vi "volumeStartInfo.vi"(6 "scan min":T3, 7 "scan max":T3, 8 "scan specification":T4={"x amplitude"=1000, "x resolution (pixels)"=28, "x offset fly-forward (iterations)"=50, "x offset fly-back (iterations)"=100, "y resolution (nr. of lines)"=80, "y step size"=30, "iterations per pixel"=5, "number of frames"=-1, "y offset (pixels)"=0, "number of y-brake lines  (before y-fly-back)"=0, "number y-brake lines (after y-fly-back)"=40, "number of y-fly-back steps"=0, "lines per z step"=1, "number of z/intensity tuples"=228, "number of repetitions (volumes or planes)"=-1, "z step size derived"=32, "choose the beginning of z scan"=FALSE, "number of frames (settings)"=80, "FPGA trajectory?"=TRUE, "Pockels cell voltage (bits)"=0, "Vy min(bits)"=0, "Vz min(bits)"=0}, 11 "derived values":T2) -> (3 "volume info":T1)   [LabVIEW 2010]
uses:
  scan_specification_cluster.ctl
  derived_values_cluster.ctl
panel:
  in  "set vol from scan settings":bool
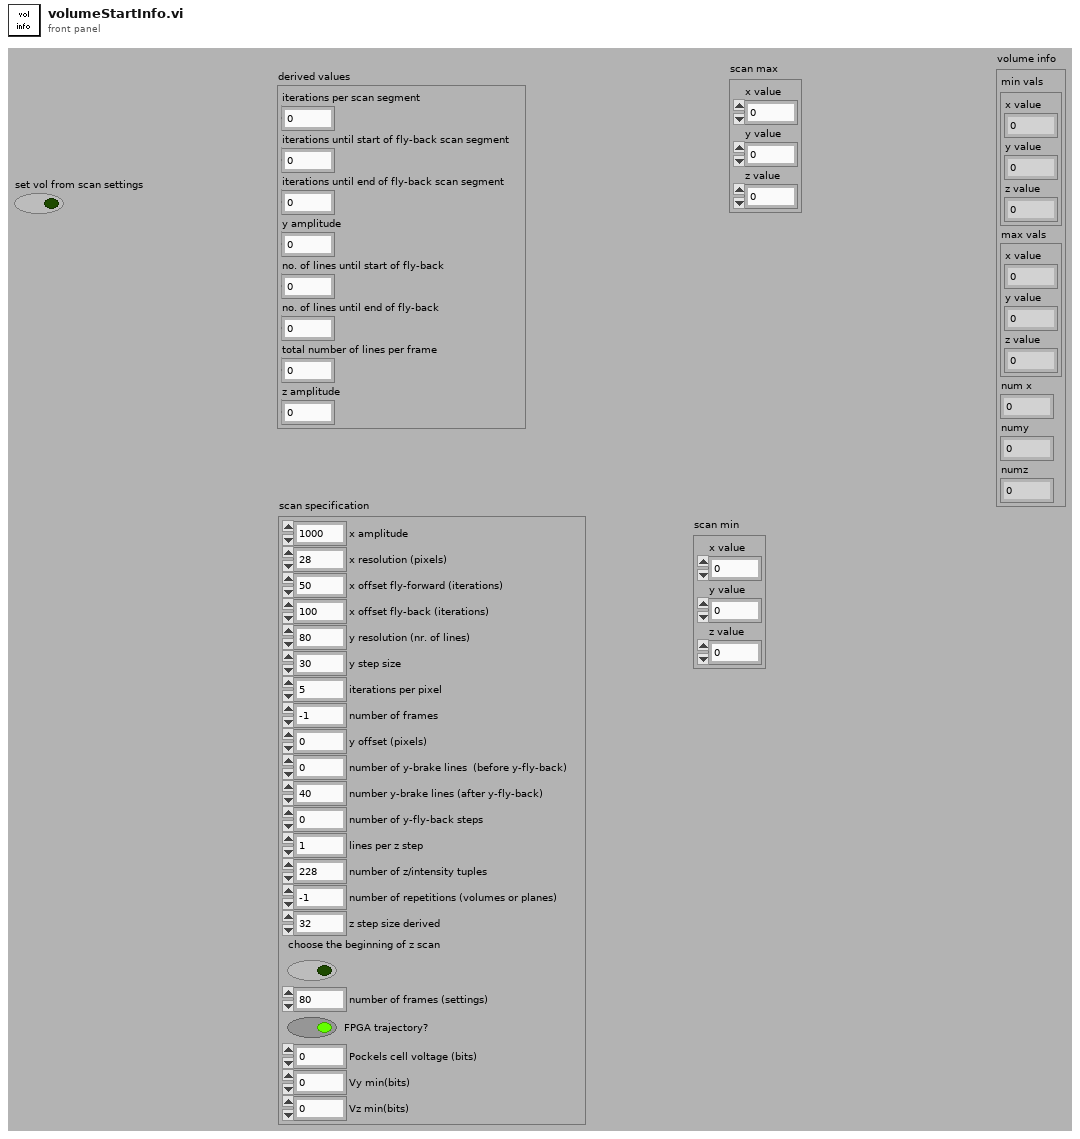
[diagram p1: front panel]
types:
  T1 = cluster{"min vals":cluster{"x value":i16, "y value":i16, "z value":i16}, "max vals":cluster{"x value":i16, "y value":i16, "z value":i16}, "num x":u32, "numy":u32, "numz":u32}
  T2 = typedef "derived_values_cluster.ctl" = cluster{"iterations per scan segment":u16, "iterations until start of fly-back scan segment":u16, "iterations until end of fly-back scan segment":u16, "y amplitude":u16, "no. of lines until start of fly-back":u16, "no. of lines until end of fly-back":u16, "total number of lines per frame ":u16, "z amplitude":u16}
  T3 = cluster{"x value":i16, "y value":i16, "z value":i16}
  T4 = typedef "scan_specification_cluster.ctl" = cluster{"x amplitude":u16, "x resolution (pixels)":u16, "x offset fly-forward (iterations)":u16, "x offset fly-back (iterations)":u16, "y resolution (nr. of lines)":u16, "y step size":u16, "iterations per pixel":u16, "number of frames":i32, "y offset (pixels)":u16, "number of y-brake lines  (before y-fly-back)":u16, "number y-brake lines (after y-fly-back)":u16, "number of y-fly-back steps":u16, "lines per z step":u16, "number of z/intensity tuples":u16, "number of repetitions (volumes or planes)":i32, "z step size derived":u16, "choose the beginning of z scan":bool, "number of frames (settings)":i32, "FPGA trajectory?":bool, "Pockels cell voltage (bits)":i16, "Vy min(bits)":i16, "Vz min(bits)":i16}
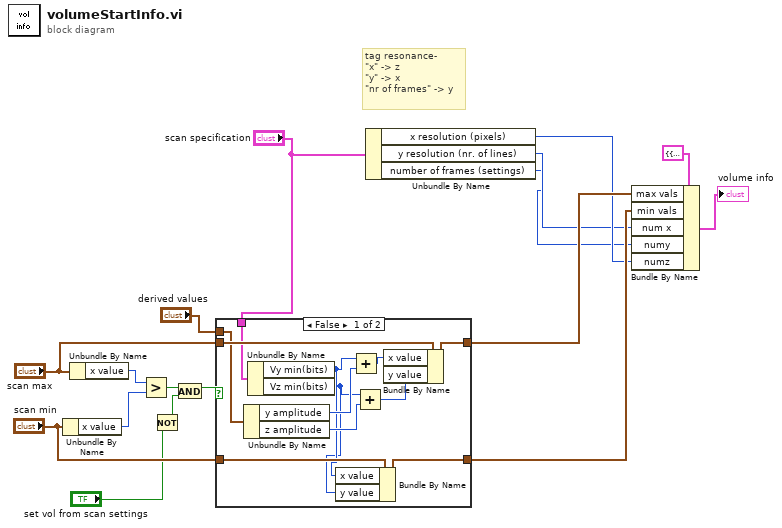
[diagram p0: block diagram]
diagram:
  # "tag resonance-\n\"x\" -> z\n\"y\" -> x\n\"nr of frames\" -> y"
  n1 = Unbundle By Name("scan min") -> ("x value"=w16:i16)
  n2 = Unbundle By Name("scan max") -> ("x value"=w17:i16)
  n3 = Greater?(x=w17, y=w16) -> (0:w3:bool)
  n4 = Not(x="set vol from scan settings") -> (.not. x?=w2:bool)
  n5 = And(x=w3, y=w2) -> (x .and. y?=w4:bool)
  n6 = case shown="False" w4 {
    tunnel: "scan max" -> [w29 w31]
    tunnel: "scan min" -> [w28 w30]
    tunnel: [w25 w31] -> w11
    tunnel: [w20 w30] -> w10
    tunnel: "derived values" -> [w27 _]
    tunnel: "scan specification" -> [w26 _]
    frame False {
      n7 = Unbundle By Name(w27) -> ("y amplitude"=w24:u16, "z amplitude"=w22:u16)
      n8 = Unbundle By Name(w26) -> ("Vy min(bits)"=w19:i16, "Vz min(bits)"=w18:i16)
      n9 = Bundle By Name(cluster=w28, "x value"=w19, "y value"=w18) -> (w20:T3)
      n10 = Add(x=w19, y=w24) -> (x+y=w23:u16)
      n11 = Add(x=w18, y=w22) -> (x+y=w21:u16)
      n12 = Bundle By Name(cluster=w29, "x value"=w23, "y value"=w21) -> (w25:T3)
    }
    frame True {
    }
  }
  n13 = Unbundle By Name("scan specification") -> ("x resolution (pixels)"=w7:u16, "y resolution (nr. of lines)"=w6:u16, "number of frames (settings)"=w5:i32)
  n14 = Bundle By Name(cluster=T1 {"min vals"={"x value"=0, "y value"=0, "z value"=0}, "max vals"={"x value"=0, "y value"=0, "z value"=0}, "num x"=0, "numy"=0, "numz"=0} ("volume info"), "max vals"=w11, "min vals"=w10, "num x"=w6, "numy"=w5, "numz"=w7) -> (→"volume info":T1)
